vi "CRYWindow WAIT WSYSTEM.vi"(10 "vi reference":refnum<vi>, 11 "sAction":string) -> (3 "sAction_Out":string)   [LabVIEW 2013]
uses:
  CRYMain Sub Window Global.vi
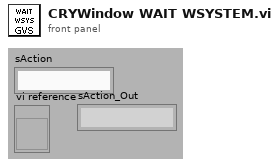
[diagram p1: front panel]
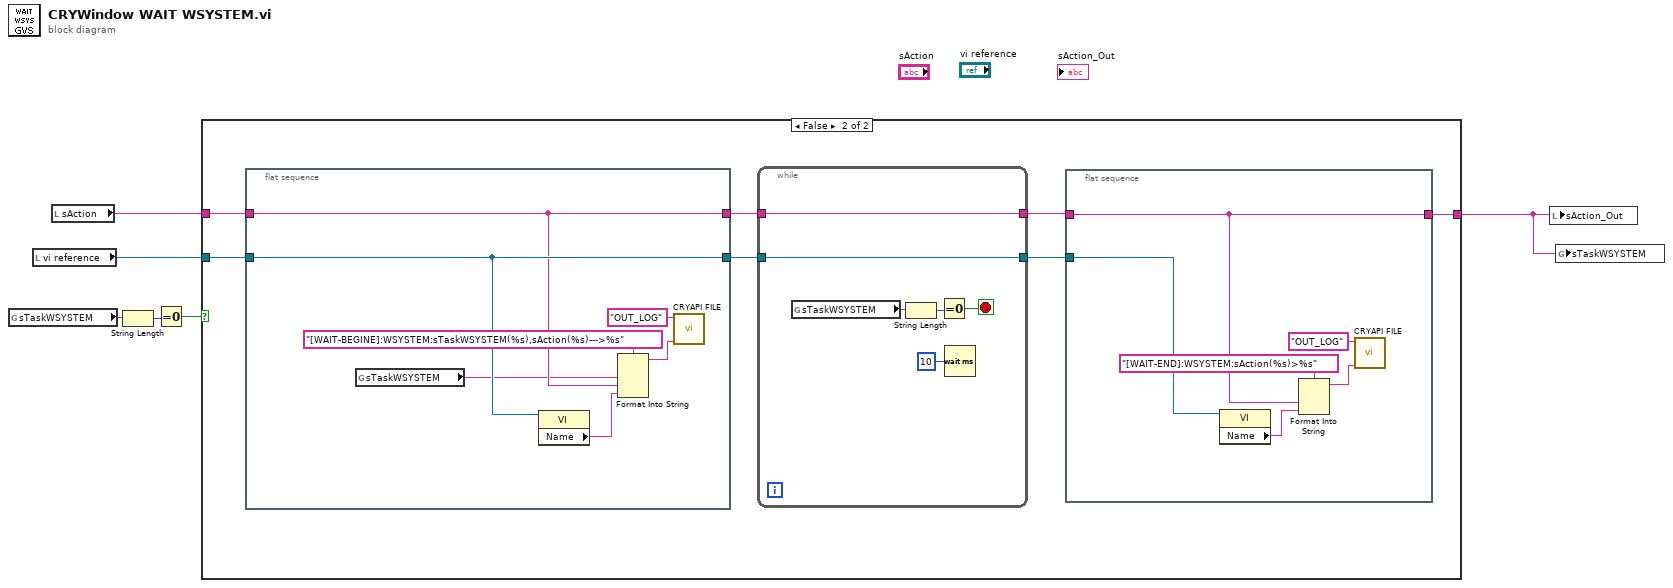
[diagram p0: block diagram]
diagram:
  n1 = global read "CRYMain Sub Window Global.vi" "sTaskWSYSTEM"() -> (w3:string)
  n2 = local read "vi reference"() -> (w5:refnum<vi>)
  n3 = local read "sAction"() -> (w6:string)
  n4 = String Length(string=w3) -> (length=w2:i32)
  n5 = Equal To 0?(x=w2) -> (x = 0?=w1:bool)
  n6 = case shown="False" w1 {
    tunnel: w6 -> [w7 w14]
    tunnel: w5 -> [_ w13]
    tunnel: [w7 w8] -> w4
    frame True {
    }
    frame False {
      n7 = flat-sequence {
        tunnel: w14 -> [w23]
        tunnel: w13 -> [w24]
        tunnel: [w23] -> w12
        tunnel: [w24] -> w10
        frame #0 {
          n8 = global read "CRYMain Sub Window Global.vi" "sTaskWSYSTEM"() -> (w21:string)
          n9 = property class="VI"(reference=w24) -> ("Name"=w22:string)  [unwired: 1 in, 2 out]
          n10 = Format Into String(format string="[WAIT-BEGINE]:WSYSTEM:sTaskWSYSTEM(%s),sAction(%s)--->%s", w21, w23, w22) -> (resulting string=w25:string)  [unwired: 2 in, 1 out]
          n11 = call "CRYAPI FILE.vi"("sData"=w25, "sAction"="OUT_LOG") -> ()  [unwired: 8 in, 2 out]
        }
      }
      n12 = while {
        tunnel: w12 -> [w31]
        tunnel: [w31] -> w11
        tunnel: w10 -> [w30]
        tunnel: [w30] -> w9
        stop <- w32 stop-if-true
        n13 = global read "CRYMain Sub Window Global.vi" "sTaskWSYSTEM"() -> (w28:string)
        n14 = String Length(string=w28) -> (length=w29:i32)
        n15 = Equal To 0?(x=w29) -> (x = 0?=w32:bool)
        n16 = Wait (ms)(milliseconds to wait=u32 10) -> ()  [unwired: 1 out]
      }
      n17 = flat-sequence {
        tunnel: w11 -> [w15]
        tunnel: [w15] -> w8
        tunnel: w9 -> [w16]
        frame #0 {
          n18 = property class="VI"(reference=w16) -> ("Name"=w20:string)  [unwired: 1 in, 2 out]
          n19 = Format Into String(format string="[WAIT-END]:WSYSTEM:sAction(%s)>%s", w15, w20) -> (resulting string=w19:string)  [unwired: 2 in, 1 out]
          n20 = call "CRYAPI FILE.vi"("sData"=w19, "sAction"="OUT_LOG") -> ()  [unwired: 8 in, 2 out]
        }
      }
    }
  }
  n21 = local write "sAction_Out"(w4) -> ()
  n22 = global write "CRYMain Sub Window Global.vi" "sTaskWSYSTEM"(w4) -> ()
